vi "Poll Until Idle.vi"(8 "error in (no error)":errorcluster, 9 "Device and Axis":string, 11 "VISA resource name":refnum<visa-resource-name>) -> (0 "error out":errorcluster, 3 "VISA resource name out":refnum<visa-resource-name>)   [LabVIEW 2013, in "Zaber A Series.lvlib"]
doc: "Waits for any movement of the device to complete and the device to be idle before continuing. To poll a specific device, use the Device and Axis input. This VI is not designed to poll all devices unless only one device is connected.\n\nThis VI requires that the Initialize VI has been called with the same serial port."
uses:
  Zaber A Series.lvlib
  Private/All Commands.ctl
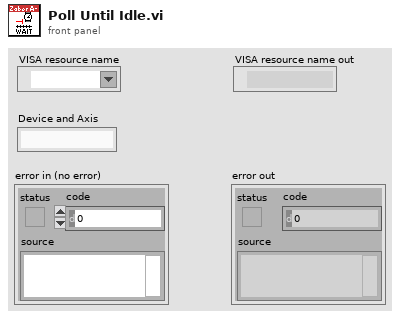
[diagram p1: front panel]
types:
  T1 = typedef "Zaber A Series.lvlib/All Commands.ctl" = string
  T2 = cluster{"Device":string, "Axis":string, "Reply Flag":string, "Status":string, "Warning Flags":string, "Data":string}[]
  T3 = cluster{"Device":string, "Axis":string, "Reply Flag":string, "Status":string, "Warning Flags":string, "Data":string}
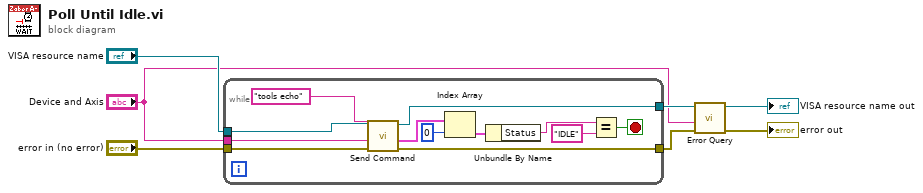
[diagram p0: block diagram]
diagram:
  n1 = while {
    tunnel: "VISA resource name" -> [w14]
    tunnel: "error in (no error)" -> [w11]
    tunnel: [w8] -> w5
    tunnel: [w10] -> w4
    tunnel: "Device and Axis" -> [w12]
    stop <- w18 stop-if-true
    n2 = call "Send Command.vi"("error in (no error)"=w11, "Device and Axis"=w12, "Command"=T1 "tools echo" ("Complete Command List"), "VISA resource name"=w14) -> ("error out"=w10:errorcluster, "Response Bundle Array"=w9:T2, "VISA resource name out"=w8:refnum<visa-resource-name>)  [unwired: 3 in, 2 out]
    n3 = Index Array(array=w9, index=0) -> (element=w15:T3)
    n4 = Unbundle By Name(w15) -> ("Status"=w17:string)
    n5 = Equal?(x=w17, y="IDLE") -> (x = y?=w18:bool)
  }
  n6 = call "Error Query.vi"("error in (no error)"=w4, "Device and Axis"="Device and Axis", "VISA resource name"=w5) -> ("error out"=→"error out":errorcluster, "VISA resource name out"=→"VISA resource name out":refnum<visa-resource-name>)  [unwired: 5 in, 2 out]
